vi "LVTimeToJSONTime.vi"(3 "LV time stamp":timestamp) -> (11 "JSON time stamp":string)   [LabVIEW 2020, in "StashRoyale.lvclass"]
uses:
  StashRoyale.lvclass
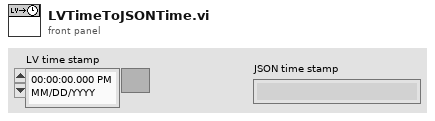
[diagram p1: front panel]
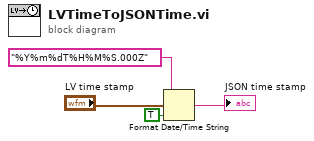
[diagram p0: block diagram]
diagram:
  n1 = Format Date/Time String(time format string (%c)="%Y%m%dT%H%M%S.000Z" ("format string"), seconds (now)="LV time stamp", UTC format=TRUE) -> (date/time string=→"JSON time stamp":string)
